vi "LabVIEW JSON Example.vi"() -> ()   [LabVIEW 2019]
doc: "Example to import or export JSON to LabVIEW Variants.\nCreated by: Ryan Pacini"
uses:
  lib/labview_json.lvlib
panel:
  out "Same?":bool
  out "Root":T1
  out "JSON":string
  in  "Root":T1={"squadName"="Super hero squad", "homeTown"="Metro City", "formed"=2016, "secretBase"="Super tower", "active"=TRUE, "members"=[{"name"="Molecule Man", "age"=29, "secretIdentity"="Dan Jukes", "powers"=["Radiation resistance", "Turning tiny", "Radiation blast"]}, {"name"="Madame Uppercut", "age"=39, "secretIdentity"="Jane Wilson", "powers"=["Million tonne punch", "Damage resistance", "Superhuman reflexes"]}, {"name"="Eternal Flame", "age"=1000000, "secretIdentity"="Unknown", "powers"=["Immortality", "Heat Immunity", "Inferno", "Teleportation", "Interdimensional travel"]}]}
  out "error out":errorcluster
  # "1. Variant to JSON"
  # "2. JSON to Variant"
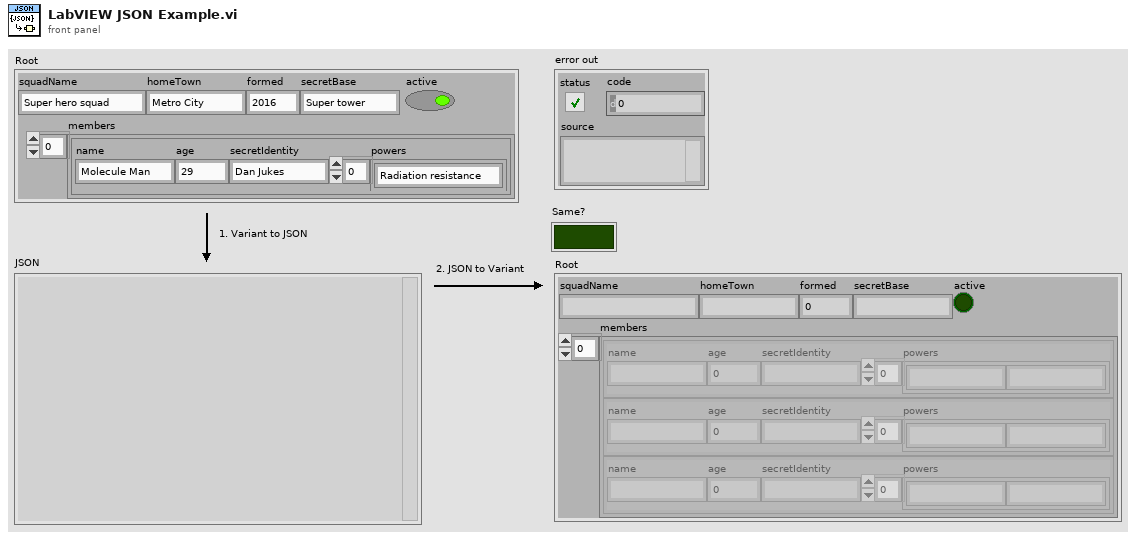
[diagram p1: front panel]
types:
  T1 = cluster{"squadName":string, "homeTown":string, "formed":i32, "secretBase":string, "active":bool, "members":cluster{"name":string, "age":i32, "secretIdentity":string, "powers":string[]}[]}
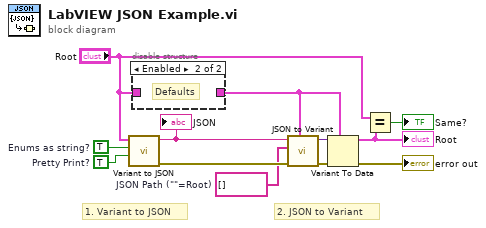
[diagram p0: block diagram]
diagram:
  w1 = string[] []  # JSON Path (""=Root)
  w8 = TRUE  # Pretty Print?
  w9 = TRUE  # Enums as string?
  # "2. JSON to Variant"
  # "1. Variant to JSON"
  n1 = call "Variant to JSON.vi"("Pretty Print? (F)"=w8, "Enums as string? (F)"=w9, "Variant in"="Root") -> ("error out"=w10:errorcluster, "JSON"=w12:string)  [unwired: 7 in]
  "JSON" <- w12
  n2 = disable-structure shown="Enabled" {
    disable-tunnel: [w13 _] -> w5
    disable-tunnel: "Root" -> [w13 _]
    frame Disabled {
    }
    frame Enabled {
      # "Defaults"
    }
  }
  n3 = call "JSON to Variant.vi"("Variant Type"=w5, "error in (no error)"=w10, "JSON Path (\"\"=Root)"=w1, "JSON"=w12) -> ("error out"=w11:errorcluster, "Variant out"=w6:variant)  [unwired: 6 in]
  n4 = Variant To Data(error in=w11, type=w5, Variant=w6) -> (data=w3:T1, error out=→"error out":errorcluster)
  "Root" <- w3
  n5 = Equal?(x="Root", y=w3) -> (x = y?=→"Same?":bool)
